vi "HFRR ADV v06 new software.vi"() -> ()   [LabVIEW 2025] (continued)
                        n2282 = local read "Set Temp"() -> (w3342:dbl)
                        n2283 = Number To Fractional String(number=w3342, precision (6)=i16 2) -> (F-format string=w3343:string)  [unwired: 2 in]
                        n2284 = Concatenate Strings("Set Temperature [deg C] :" ("Content"), w3343) -> (w3345:string)
                        n2285 = local read "EVENT LOG"() -> (w3347:string)
                        n2286 = call "Event Log.vi"("Content"=w3345, "EVENT LOG"=w3347) -> ("EVENT LOG"=w3346:string)  [unwired: 8 in, 1 out]
                        n2287 = local write "EVENT LOG"(w3346) -> ()
                      }
                      frame #28 {
                        n2288 = Wait (ms)(milliseconds to wait=u32 50) -> ()  [unwired: 1 out]
                      }
                      frame #29 {
                        n2289 = local read "Set Rh"() -> (w3350:dbl)
                        n2290 = Number To Fractional String(number=w3350, precision (6)=i16 2) -> (F-format string=w3351:string)  [unwired: 2 in]
                        n2291 = Concatenate Strings("Set Humidity [%RH] :" ("Content"), w3351) -> (w3353:string)
                        n2292 = local read "EVENT LOG"() -> (w3355:string)
                        n2293 = call "Event Log.vi"("Content"=w3353, "EVENT LOG"=w3355) -> ("EVENT LOG"=w3354:string)  [unwired: 8 in, 1 out]
                        n2294 = local write "EVENT LOG"(w3354) -> ()
                      }
                      frame #30 {
                        n2295 = Wait (ms)(milliseconds to wait=u32 50) -> ()  [unwired: 1 out]
                      }
                      frame #31 {
                        n2296 = local read "test time"() -> (w3358:dbl)
                        n2297 = Number To Fractional String(number=w3358, precision (6)=i16 1) -> (F-format string=w3359:string)  [unwired: 2 in]
                        n2298 = Concatenate Strings("Test Duration [mins] :" ("Content"), w3359) -> (w3361:string)
                        n2299 = local read "EVENT LOG"() -> (w3363:string)
                        n2300 = call "Event Log.vi"("Content"=w3361, "EVENT LOG"=w3363) -> ("EVENT LOG"=w3362:string)  [unwired: 8 in, 1 out]
                        n2301 = local write "EVENT LOG"(w3362) -> ()
                      }
                      frame #32 {
                        w3364 = dbl[] [] ("History Data")
                        w3365 = cluster{"y":dbl, dbl, "y":dbl}[] [] ("History Data")
                        w3366 = FALSE ("Visible")
                        n2302 = property on="Stroke ( mm )" class="WFChart (strict)"("History Data"=w3365) -> ()  [unwired: 2 in, 2 out]
                        n2303 = property on="Humidity ( %RH )" class="WFChart (strict)"("History Data"=w3364) -> ()  [unwired: 2 in, 2 out]
                        n2304 = property on="Temperature ( Deg C )" class="WFChart (strict)"("History Data"=w3364) -> ()  [unwired: 2 in, 2 out]
                        n2305 = property on="Electrical Contact Resistance ( % )" class="WFChart (strict)"("History Data"=w3364) -> ()  [unwired: 2 in, 2 out]
                        n2306 = property on="Coefficient of Friction" class="WFChart (strict)"("History Data"=w3364) -> ()  [unwired: 2 in, 2 out]
                        n2307 = property on="Frictional Force ( N )" class="WFChart (strict)"("History Data"=w3364) -> ()  [unwired: 2 in, 2 out]
                        n2308 = property on="Coefficient of Friction" class="WFChart (strict)"("History Data"=w3364) -> ()  [unwired: 2 in, 2 out]
                        n2309 = property on="Frictional Force ( N )" class="WFChart (strict)"("History Data"=w3364) -> ()  [unwired: 2 in, 2 out]
                        n2310 = property on="Electrical Contact Resistance ( % )" class="WFChart (strict)"("History Data"=w3364) -> ()  [unwired: 2 in, 2 out]
                        n2311 = property on="Humidity ( %RH )" class="WFChart (strict)"("History Data"=w3364) -> ()  [unwired: 2 in, 2 out]
                        n2312 = property on="Stroke ( mm )" class="WFChart (strict)"("History Data"=w3365) -> ()  [unwired: 2 in, 2 out]
                        n2313 = property on="Temperature ( Deg C )" class="WFChart (strict)"("History Data"=w3364) -> ()  [unwired: 2 in, 2 out]
                        n2314 = property on="Service Password Log" class="Str"("Visible"=w3366) -> ()  [unwired: 2 in, 2 out]
                        n2315 = property on="Password 3" class="Clust (strict)"("Visible"=w3366) -> ()  [unwired: 2 in, 2 out]
                      }
                    }
                    "TEST FILE NAM,E SAVED" <- TRUE ("TEST FILE NAM,E SAVED")
                  }
                }
              }
            }
          }
        }
        n2316 = case shown="True" w2670 {
          frame False {
            n2317 = local write "tfalg"(0.0 ("tfalg")) -> ()
          }
          frame True {
            n2318 = local read "tfalg"() -> (w2815:dbl)
            n2319 = Equal?(x=w2815, y=0.0) -> (x = y?=w2816:bool)
            n2320 = case shown="True" w2816 {
              frame False {
              }
              frame True {
                n2321 = local read "Total No. of Tests"() -> (w2819:dbl)
                n2322 = local write "tfalg"(1.0 ("tfalg")) -> ()
                n2323 = local write "acq 2"(FALSE ("acq 2")) -> ()
                n2324 = Wait (ms)(milliseconds to wait=u32 200) -> ()  [unwired: 1 out]
                n2325 = Increment(x=w2819) -> (x+1=w2818:dbl)
                n2326 = local write "Total No. of Tests"(w2818) -> ()
              }
            }
          }
        }
        n2327 = local write "Test \nStatus"(w2676) -> ()
        n2328 = local write "Save"(w2676) -> ()
        n2329 = local read "Main Tab"() -> (w2633:T2)
        n2330 = case shown="True" w2657 {
          tunnel: [FALSE ("RUN") TRUE ("RUN")] -> w2656
          tunnel: [_ 1] -> w2649
          frame False {
          }
          frame True {
          }
        }
        n2331 = In Range and Coerce(upper limit=w2664, x=w2637, lower limit=w2663) -> (In Range?=w2655:bool)  [unwired: 1 out]
        n2332 = In Range and Coerce(upper limit=w2661, x=w2636, lower limit=w2662) -> (In Range?=w2653:bool)  [unwired: 1 out]
        n2333 = case shown="True" w2669 {
          frame False {
            n2334 = local read "Rt 3"() -> (w2797:bool)
            n2335 = case shown="True" w2797 {
              frame False {
              }
              frame True {
                n2336 = local write "Rt 3"(FALSE ("Rt 3")) -> ()
                n2337 = local write "Json End Flg"(TRUE ("Upld AR 2")) -> ()
              }
            }
            "Rt" <- TRUE ("Rt")
            "Rt 2" <- FALSE ("Rt")
          }
          frame True {
            n2338 = local read "Rt"() -> (w2804:bool)
            n2339 = local write "Rt 2"(TRUE ("Rt 2")) -> ()
            n2340 = case shown="True" w2804 {
              frame False {
              }
              frame True {
                w2805 = TRUE ("Upld AR 2")
                n2341 = local write "Rt"(FALSE ("Rt")) -> ()
                n2342 = local write "Upld AR"(w2805) -> ()
                n2343 = local write "Json St Flg"(w2805) -> ()
              }
            }
            "Rt 3" <- TRUE ("Rt 3")
          }
        }
        n2344 = case shown="True" w2655 {
          tunnel: [FALSE ("RUN") TRUE ("RUN")] -> w2654
          tunnel: [_ 2] -> w2648
          frame False {
          }
          frame True {
          }
        }
        n2345 = case shown="True" w2653 {
          tunnel: [FALSE ("RUN") TRUE ("RUN")] -> w2652
          tunnel: [_ 3] -> w2647
          frame False {
          }
          frame True {
          }
        }
        n2346 = case shown="\"Acquire\"" w2633 {
          tunnel: w2635 -> [_ w2866]
          frame Default {
            w2865 = 0.0 ("output")
            n2347 = local write "PID-out"(w2865) -> ()
            n2348 = local write "Frequency ( Hz )"(w2865) -> ()
          }
          frame "Acquire" {
            n2349 = stacked-sequence {
              frame #0 {
                n2350 = local read "Auto Start Test"() -> (w2868:bool)
                n2351 = case shown="True" w2868 {
                  tunnel: "RUN" -> [w2889 w2892]
                  tunnel: [w2889 w2891] -> w2869
                  frame False {
                  }
                  frame True {
                    n2352 = local read "Auto Start Temp"() -> (w2890:bool)
                    n2353 = Or(x=w2892, y=w2890) -> (x .or. y?=w2891:bool)
                  }
                }
                n2354 = local read "clk"() -> (w2888:dbl)
                n2355 = local read "Save"() -> (w2884:bool)
                n2356 = Equal?(x=w2888, y=0.0) -> (x = y?=w2885:bool)
                n2357 = And(x=w2885, y=w2884) -> (x .and. y?=w2886:bool)
                n2358 = Not(x="Engage") -> (.not. x?=w2875:bool)
                n2359 = case shown="False" w2869 {
                  tunnel: [0.0 w2910] -> w2871
                  frame False {
                    (unwired) TRUE ("Visible")
                    n2360 = local read "Auto Start Test"() -> (w2896:bool)
                    n2361 = local write "Start Time"(TRUE ("Start Time")) -> ()
                    n2362 = property on="Stroke 2" class="DigNum (strict)"("Visible"=FALSE) -> ()  [unwired: 2 in, 2 out]
                    n2363 = case shown="False" w2896 {
                      frame False {
                        n2364 = property on="Heater Button" class="Bool (strict)"("DisabledEnum"=T13."Enabled" ("Disabled")) -> ()  [unwired: 2 in, 2 out]
                        n2365 = property on="Humidity" class="Bool (strict)"("DisabledEnum"=T13."Enabled" ("Disabled")) -> ()  [unwired: 2 in, 2 out]
                      }
                      frame True {
                      }
                    }
                    n2366 = case shown="False" "TestCompFlg" {
                      frame False {
                        n2367 = local read "StartFlg"() -> (w2904:bool)
                        n2368 = case shown="True" w2904 {
                          frame False {
                          }
                          frame True {
                            n2369 = flat-sequence {
                              frame #0 {
                                n2370 = local read "EVENT LOG"() -> (w2906:string)
                                n2371 = call "Event Log.vi"("Content"="Test was interrupted", "EVENT LOG"=w2906) -> ("EVENT LOG"=w2907:string)  [unwired: 8 in, 1 out]
                                n2372 = local write "EVENT LOG"(w2907) -> ()
                              }
                              frame #1 {
                                w2909 = FALSE ("StartFlg")
                                n2373 = property on="Heater Button" class="Bool (strict)"("Val(Sgnl)"=FALSE ("Value (Signaling)")) -> ()  [unwired: 2 in, 2 out]
                                n2374 = local write "Heater Button"(w2909) -> ()
                                n2375 = local write "StartFlg"(w2909) -> ()
                                n2376 = local write "Humidity"(w2909) -> ()
                              }
                            }
                          }
                        }
                      }
                      frame True {
                      }
                    }
                    n2377 = local write "String 14"("Test will autostart once parameters reach the set value." ("String 14")) -> ()
                  }
                  frame True {
                    (unwired) FALSE ("Visible")
                    n2378 = property on="Stroke 2" class="DigNum (strict)"("Visible"=TRUE) -> ()  [unwired: 2 in, 2 out]
                    n2379 = property on="STOP 2" class="Bool (strict)"("Disabled"=u8 2) -> ()  [unwired: 2 in, 2 out]
                    n2380 = local write "String 14"(" Running....." ("String 14")) -> ()
                    n2381 = property on="Heater Button" class="Bool (strict)"("DisabledEnum"=T13."Disabled and Grayed Out" ("Disabled")) -> ()  [unwired: 2 in, 2 out]
                    n2382 = property on="Humidity" class="Bool (strict)"("DisabledEnum"=T13."Disabled and Grayed Out" ("Disabled")) -> ()  [unwired: 2 in, 2 out]
                    n2383 = case shown="True" "Start Time" {
                      selector: "Start Time" -> [_ w2929]
                      frame False {
                      }
                      frame True {
                        n2384 = Not(x=w2929) -> (.not. x?=w2928:bool)
                        n2385 = local write "Start Time"(w2928) -> ()
                        n2386 = local read "EVENT LOG"() -> (w2930:string)
                        n2387 = call "Event Log.vi"("Content"="Test in progress", "EVENT LOG"=w2930) -> ("EVENT LOG"=w2932:string)  [unwired: 8 in, 1 out]
                        n2388 = local write "EVENT LOG"(w2932) -> ()
                      }
                    }
                    n2389 = disable-structure shown="Enabled" {
                      disable-tunnel: [w2921 w2927] -> w2910
                      frame Disabled {
                        n2390 = local read "Set Hz"() -> (w2924:dbl)
                        n2391 = call <vilib>:"Uniform White Noise Waveform.vi"() -> ("signal out"=w2923:waveform(dbl))  [unwired: 10 in, 1 out]
                        n2392 = Random Number (0-1)() -> (number: 0 to 1=w2920:dbl)
                        n2393 = Add(x=w2924, y=w2923) -> (x+y=w2922:waveform(dbl))
                        n2394 = Multiply(x=ext 0.01 ("y"), y=w2920) -> (x*y=w2918:ext)
                        n2395 = Multiply(x=w2922, y=w2918) -> (x*y=w2921:waveform(ext))
                      }
                      frame Enabled {
                        n2396 = call-poly <vilib>:"Random Number (Range).vi"("lower bound (0)"=49.5, "upper bound (100)"=50.5) -> ("number"=w2927:dbl)  [unwired: 9 in]
                      }
                    }
                    "StartFlg" <- TRUE ("StartFlg")
                  }
                }
                n2397 = case shown="True" w2886 {
                  frame False {
                  }
                  frame True {
                    n2398 = local write "clk"(10.0 ("clk")) -> ()
                    n2399 = Get Date/Time In Seconds() -> (seconds since 1Jan1904=w2935:timestamp)
                    n2400 = To Double Precision Float(number=w2935) -> (double precision float=w2933:dbl)
                    n2401 = local write "acq timer"(w2933) -> ()
                    n2402 = local write "act save time"(w2933) -> ()
                  }
                }
                n2403 = call "Elapsed Time"("Time Target (s)"="Countdown", "Reset"=w2875) -> ("Elapsed Time (s)"=w2880:dbl, "Time has Elapsed"=w2878:bool)  [unwired: 10 in, 6 out]
                "Countdown 2" <- w2880
                n2404 = Subtract(x=w2880, y=2.0) -> (x-y=w2883:dbl)
                n2405 = Less?(x=w2883, y="Countdown") -> (x < y?=w2881:bool)
                n2406 = And(x=w2881, y=w2878) -> (x .and. y?=w2877:bool)
                n2407 = case shown="True" w2877 {
                  frame False {
                  }
                  frame True {
                    (unwired) dbl[] [] ("History Data")
                    n2408 = local write "Engage"(FALSE ("Engage")) -> ()
                    n2409 = local write "RUN"(TRUE ("RUN")) -> ()
                    n2410 = local read "Humidity ( %RH )"() -> (→"Rh Before":dbl)
                  }
                }
                n2411 = local read "Test \nStatus"() -> (w2873:bool)
                n2412 = Select(t=w2871, s=w2873, f=0.0) -> (s? t:f=w2872:dbl)
                n2413 = local write "Frequency ( Hz )"(w2872) -> ()
              }
              frame #1 {
                w2958 = 1000000.0 ("x")
                # "HC;1/0\nST;VALUE"
                # "Elapsed time\ncof\nstroke\nAir temp\nTemp\nHumidity"
                # "acq timer\n\nact save time"
                # "convert to microseconds"
                n2414 = local read "COUNT"() -> (w2941:i32)
                n2415 = local read "Rate"() -> (w2954:dbl)
                n2416 = Divide(x=w2958, y=w2954) -> (x/y=w2959:dbl)
                n2417 = Greater Or Equal?(x=w2941, y=250) -> (x >= y?=w2940:bool)
                n2418 = Get Date/Time In Seconds() -> (seconds since 1Jan1904=w2961:timestamp)
                n2419 = case shown="True" w2940 {
                  frame False {
                    n2420 = local read "COUNT"() -> (w2962:i32)
                    n2421 = Increment(x=w2962) -> (x+1=w2963:i32)
                    n2422 = local write "COUNT"(w2963) -> ()
                  }
                  frame True {
                    n2423 = local write "COUNT"(0 ("COUNT")) -> ()
                  }
                }
                n2424 = local read "Samplingtime 2"() -> (w2939:dbl)
                n2425 = local read "act save time"() -> (w2956:dbl)
                n2426 = Divide(x=w2959, y=w2958) -> (x/y=w2957:dbl)
                n2427 = To Double Precision Float(number=w2961) -> (double precision float=w2950:dbl)
                n2428 = Add(x=w2956, y=w2939) -> (x+y=w2955:dbl)
                n2429 = local read "acq timer"() -> (w2960:dbl)
                n2430 = local read "COUNT"() -> (w2943:i32)
                n2431 = Greater Or Equal?(x=w2950, y=w2955) -> (x >= y?=w2938:bool)
                n2432 = Multiply(x=w2957, y=w2943) -> (x*y=w2949:dbl)
                n2433 = Subtract(x=w2950, y=w2960) -> (x-y=w2952:dbl)
                n2434 = local read "Save"() -> (w2953:bool)
                n2435 = Add(x=w2952, y=w2949) -> (x+y=w2936:dbl)
                "Elapsed time 3" <- w2936
                n2436 = And(x=w2938, y=w2953) -> (x .and. y?=w2951:bool)
                n2437 = Divide(x=w2936, y=60.0) -> (x/y=w2947:dbl)
                n2438 = local read "Test \nStatus"() -> (w2937:bool)
                n2439 = local read "clk"() -> (w2944:dbl)
                n2440 = Equal?(x=w2944, y=10.0) -> (x = y?=w2946:bool)
                n2441 = case shown="True" w2951 {
                  tunnel: w2950 -> [_ w3072]
                  tunnel: [FALSE ("Boolean 2") TRUE ("Boolean 2")] -> _
                  frame False {
                  }
                  frame True {
                    w3026 = ";" ("Substring")
                    # "Pid out/\nFreq response value"
                    n2442 = local write "act save time"(w3072) -> ()
                    n2443 = local read "FILE"() -> (w3020:string)
                    n2444 = call "file check.vi"("file name in"=w3020) -> ("error out"=w3023:errorcluster, "file name out"=w3018:string)  [unwired: 9 in]
                    n2445 = call "FILE PATH CREATION.vi"("error in"=w3023, "FILE NAME :"=w3018) -> ("FILE OUT"=w3021:path)  [unwired: 8 in, 1 out]
                    n2446 = Concatenate Strings(w3018, ".dgf" ("Substring")) -> (w3022:string)
                    n2447 = local read "FF 2"() -> (→"Frictional Force ( N )" →"Frictional Force ( N )":dbl)
                    n2448 = Build Path(base path=w3021, name or relative path=w3022) -> (appended path=w3017:path)
                    n2449 = local read "COF 2"() -> (w3031:dbl)
                    "cof" <- w3031
                    "Coefficient of Friction" <- w3031
                    "COF 4" <- w3031
                    "Coefficient of Friction" <- w3031
                    n2450 = local read "LVDT STROKE"() -> (w3015:dbl)
                    n2451 = local read "Add up Stroke"() -> (w3013:dbl)
                    n2452 = local read "TEMP"() -> (w3034:dbl)
                    "Temp" <- w3034
                    "Temperature ( Deg C )" <- w3034
                    n2453 = local read "Humidity ( %RH )"() -> (w3033:dbl)
                    "Humidity ( %RH )" <- w3033
                    "Humidity ( %RH )" <- w3033
                    n2454 = local read "Frequency ( Hz )"() -> (w3040:dbl)
                    n2455 = local read "Elapsed time"() -> (w3065:dbl)
                    n2456 = local read "AIR TEMP"() -> (w3038:dbl)
                    n2457 = local read "PID-out"() -> (w3043:dbl)
                    n2458 = Subtract(x=w3015, y=w3013) -> (x-y=w3014:dbl)
                    n2459 = Absolute Value(x=w3014) -> (abs(x)=w3012:dbl)
                    n2460 = local write "Temperature ( Deg C )"(w3034) -> ()
                    n2461 = Number To Fractional String(number=w3012, width (-)=i16 9 ("precision (6)"), precision (6)=i16 6) -> (F-format string=w3058:string)  [unwired: 1 in]
                    n2462 = Number To Fractional String(number=w3038, width (-)=i16 9 ("precision (6)"), precision (6)=i16 3) -> (F-format string=w3057:string)  [unwired: 1 in]
                    n2463 = Number To Fractional String(number=w3034, width (-)=i16 9 ("precision (6)"), precision (6)=i16 3) -> (F-format string=w3054:string)  [unwired: 1 in]
                    n2464 = Number To Fractional String(number=w3033, width (-)=i16 9 ("precision (6)"), precision (6)=i16 3) -> (F-format string=w3051:string)  [unwired: 1 in]
                    n2465 = Number To Fractional String(number=0.0, width (-)=i16 9 ("precision (6)"), precision (6)=i16 3) -> (F-format string=w3048:string)  [unwired: 1 in]
                    n2466 = Number To Fractional String(number=w3043, width (-)=i16 9 ("precision (6)"), precision (6)=i16 3) -> (F-format string=w3044:string)  [unwired: 1 in]
                    n2467 = Number To Fractional String(number=w3040, width (-)=i16 9 ("precision (6)"), precision (6)=i16 3) -> (F-format string=w3039:string)  [unwired: 1 in]
                    n2468 = Number To Fractional String(number=w3031, width (-)=i16 9 ("precision (6)"), precision (6)=i16 6) -> (F-format string=w3066:string)  [unwired: 1 in]
                    n2469 = Number To Fractional String(number=w3065, width (-)=i16 14 ("precision (6)"), precision (6)=i16 3) -> (F-format string=w3067:string)  [unwired: 1 in]
                    n2470 = Bundle("y"=1.02, w3012, "y"=0.98) -> (w3032:cluster{"y":dbl, dbl, "y":dbl})  [unwired: 1 in]
                    n2471 = Number To Fractional String(number="Ambient Humidity :", width (-)=i16 9 ("precision (6)"), precision (6)=i16 6) -> (F-format string=w3024:string)  [unwired: 1 in]
                    n2472 = local read "RUN"() -> (w3030:bool)
                    n2473 = case shown="True" w3030 {
                      tunnel: w3032 -> [_ w3077]
                      tunnel: w3012 -> [_ w3076]
                      tunnel: w3012 -> [_ w3074]
                      tunnel: w3012 -> [_ w3075]
                      frame False {
                      }
                      frame True {
                        "Stroke ( mm )" <- w3077
                        "Stroke ( mm )" <- w3077
                        "Stroke 4" <- w3076
                        "Stroke 3" <- w3074
                        "Stroke 2" <- w3075
                        "measured_stroke" <- w3074
                      }
                    }
                    n2474 = Concatenate Strings(w3067, w3026, w3066, w3026, w3058, w3026, w3057, w3026, w3054, w3026, w3051, w3026, w3048, w3026, w3044, w3026, w3039, w3026, w3024, "\r") -> (w3064:string)
                    n2475 = call <vilib>:"Write Characters To File.vi"("append to file? (new file:F)"=TRUE, "character string"=w3064, "file path (dialog if empty)"=w3017) -> ()  [unwired: 2 in, 1 out]
                    "refresh flag" <- TRUE ("refresh flag")
                  }
                }
                n2476 = case shown="True" w2937 {
                  tunnel: w2947 -> [_ w2973]
                  tunnel: w2952 -> [_ w2983]
                  tunnel: [0.0 w2979] -> _
                  tunnel: w2946 -> [_ w2978]
                  tunnel: [0.0 w2977] -> _
                  tunnel: w2936 -> [_ w2977]
                  tunnel: w2950 -> [w2966 _]
                  frame False {
                    n2477 = local write "acq timer"(w2966) -> ()
                    n2478 = local write "Test Duration Status"(0.0 ("Test Duration Status")) -> ()
                  }
                  frame True {
                    n2479 = local read "Set Hz"() -> (w2980:dbl)
                    n2480 = local write "Elapsed time"(w2973) -> ()
                    n2481 = local read "test time"() -> (w2972:dbl)
                    n2482 = Multiply(x=w2983, y=w2980) -> (x*y=w2982:dbl)
                    n2483 = case shown="False" w2978 {
                      tunnel: w2982 -> [w2984 _]
                      tunnel: [w2984 1.0] -> w2979
                      frame False {
                        n2484 = local write "Cycles elapsed"(w2984) -> ()
                      }
                      frame True {
                      }
                    }
                    n2485 = Greater?(x=w2973, y=w2972) -> (0:w2981:bool)
                    n2486 = Subtract(x=w2972, y=w2973) -> (x-y=w2971:dbl)
                    "time" <- w2971
                    n2487 = Multiply(x=w2971, y=60.0) -> (x*y=w2970:dbl)
                    n2488 = local write "Time Remaining"(w2970) -> ()
                    n2489 = local write "Remaining Time"(w2970) -> ()
                    n2490 = case shown="True" w2981 {
                      frame False {
                      }
                      frame True {
                        n2491 = stacked-sequence {
                          frame #0 {
                            w2989 = T13."Enabled" ("Disabled")
                            w2988 = FALSE ("TEST FILE NAM,E SAVED")
                            w2990 = "" ("FILE")
                            w2991 = TRUE ("Visible")
                            n2492 = local write "Humidity"(FALSE ("Humidity")) -> ()
                            n2493 = local write "RUN"(FALSE ("OK Button 2")) -> ()
                            n2494 = local write "Heater Button"(FALSE ("Heater Button")) -> ()
                            n2495 = local write "Auto Start Test"(FALSE ("Auto Start Test")) -> ()
                            n2496 = local write "TestCompFlg"(TRUE ("StpFlg")) -> ()
                            n2497 = local read "Humidity ( %RH )"() -> (→"Rh After":dbl)
                            n2498 = property on="STOP 2" class="Bool (strict)"("Disabled"=u8 0) -> ()  [unwired: 2 in, 2 out]
                            n2499 = local read "EVENT LOG"() -> (w2996:string)
                            n2500 = call "Event Log.vi"("Content"="Test Completed", "EVENT LOG"=w2996) -> ("EVENT LOG"=w2995:string)  [unwired: 8 in, 1 out]
                            n2501 = property on="RUN" class="Bool (strict)"("Visible"=w2991) -> ()  [unwired: 2 in, 2 out]
                            n2502 = property on="Auto Start Test" class="Bool (strict)"("Visible"=w2991) -> ()  [unwired: 2 in, 2 out]
                            n2503 = local write "Batch Ref Num :"(w2990) -> ()
                            n2504 = local write "FILE"(w2990) -> ()
                            n2505 = local write "EVENT LOG"(w2995) -> ()
                            n2506 = local write "TEST FILE NAM,E SAVED"(w2988) -> ()
                            n2507 = local write "Fuel Discription :"(w2990) -> ()
                            n2508 = local write "START TEMP"(w2988) -> ()
                            n2509 = local write "Remarks :"(w2990) -> ()
                            n2510 = local write "Main Dashboard Buttons"(T1."Imaging" ("Main Dashboard Buttons")) -> ()
                            n2511 = local write "Main Tab"(T2."Adv Scar" ("Main Tab")) -> ()
                            n2512 = property on="FRICVALZ 2" class="Bool (strict)"("DisabledEnum"=w2989) -> ()  [unwired: 2 in, 2 out]
                            n2513 = property on="FRICVALZ 3" class="Bool (strict)"("DisabledEnum"=w2989) -> ()  [unwired: 2 in, 2 out]
                            n2514 = property on="FRICVALZ 4" class="Bool (strict)"("DisabledEnum"=w2989) -> ()  [unwired: 2 in, 2 out]
                          }
                          frame #1 {
                            n2515 = Wait (ms)(milliseconds to wait=u32 1500) -> ()  [unwired: 1 out]
                          }
                          frame #2 {
                            n2516 = local write "Command"("VC;0") -> ()
                          }
                          frame #3 {
                            n2517 = Wait (ms)(milliseconds to wait=u32 1500) -> ()  [unwired: 1 out]
                          }
                          frame #4 {
                            n2518 = local write "Command"("VC;0") -> ()
                          }
                          frame #5 {
                            n2519 = Wait (ms)(milliseconds to wait=u32 1500) -> ()  [unwired: 1 out]
                          }
                          frame #6 {
                            n2520 = local write "Command"("ST;0") -> ()
                          }
                          frame #7 {
                            n2521 = local write "measured_stroke"(0.0 ("measured_stroke")) -> ()
                            n2522 = Wait (ms)(milliseconds to wait=u32 1500) -> ()  [unwired: 1 out]
                          }
                          frame #8 {
                            n2523 = local write "Command"("HE;0") -> ()
                          }
                        }
                      }
                    }
                    n2524 = Divide(x=w2973, y=w2972) -> (x/y=w2976:dbl)
                    n2525 = Multiply(x=w2976, y=100.0) -> (x*y=w2974:dbl)
                    n2526 = local write "Test Duration Status"(w2974) -> ()
                  }
                }
              }
              frame #2 {
                n2527 = case shown="True" "Heater Button" {
                  tunnel: [0.0 ("output") w3100] -> w3078
                  frame False {
                    w3081 = TRUE ("tmpchk")
                    n2528 = local read "TEMP"() -> (w3082:dbl)
                    n2529 = local write "Temp ini"(w3082) -> ()
                    n2530 = local write "Reset 4"(w3081) -> ()
                    n2531 = local write "tmpchk"(w3081) -> ()
                    n2532 = local write "reinit"(TRUE ("reinit")) -> ()
                    n2533 = local write "manual temp log"(TRUE ("manual temp log")) -> ()
                  }
                  frame True {
                    # "Logic to turn off\nthe heater when \ntemp is not rising.\nTime - 60 sec\nDelta t- 5°c"
                    n2534 = local read "Temp ini"() -> (w3089:dbl)
                    n2535 = local read "Auto Start Test"() -> (w3085:bool)
                    n2536 = Less?(x=w3089, y=53.0) -> (x < y?=w3087:bool)
                    n2537 = case shown="False" w3085 {
                      frame False {
                        n2538 = local read "Set Temp"() -> (w3109:dbl)
                        n2539 = local read "TEMP"() -> (w3108:dbl)
                        n2540 = Subtract(x=w3109, y=w3108) -> (x-y=w3107:dbl)
                        n2541 = Absolute Value(x=w3107) -> (abs(x)=w3106:dbl)
                        n2542 = Less?(x=w3106, y=0.5) -> (x < y?=w3104:bool)
                        n2543 = case shown="True" w3104 {
                          tunnel: "manual temp log" -> [_ w3110]
                          frame False {
                          }
                          frame True {
                            n2544 = case shown="True" w3110 {
                              selector: w3110 -> [_ w3111]
                              frame False {
                              }
                              frame True {
                                # "#Event log"
                                n2545 = Not(x=w3111) -> (.not. x?=w3112:bool)
                                n2546 = local write "manual temp log"(w3112) -> ()
                                n2547 = local read "EVENT LOG"() -> (w3115:string)
                                n2548 = call "Event Log.vi"("Content"="Target Temperature reached", "EVENT LOG"=w3115) -> ("EVENT LOG"=w3114:string)  [unwired: 8 in, 1 out]
                                n2549 = local write "EVENT LOG"(w3114) -> ()
                              }
                            }
                          }
                        }
                      }
                      frame True {
                        n2550 = local write "manual temp log"(TRUE ("manual temp log")) -> ()
                      }
                    }
                    n2551 = And(x="tmpchk", y=w3087) -> (x .and. y?=w3090:bool)
                    n2552 = case shown="True" w3090 {
                      frame False {
                      }
                      frame True {
                        n2553 = call "Elapsed Time8"("Time Target (s)"=300.0, "Reset"="Reset 4") -> ("Time has Elapsed"=w3117:bool)  [unwired: 10 in, 7 out]
                        n2554 = flat-sequence {
                          tunnel: w3117 -> [_]
                          frame #0 {
                            n2555 = local write "Reset 4"(FALSE ("Reset 4")) -> ()
                          }
                        }
                        n2556 = case shown="True" w3117 {
                          frame False {
                          }
                          frame True {
                            n2557 = local read "Temp ini"() -> (w3124:dbl)
                            n2558 = Add(x=w3124, y=5.0) -> (x+y=w3122:dbl)
                            n2559 = local read "TEMP"() -> (w3125:dbl)
                            n2560 = Greater?(x=w3125, y=w3122) -> (0:w3123:bool)
                            n2561 = case shown="False" w3123 {
                              frame False {
                                n2562 = local write "Heater Button"(FALSE ("Heater Button")) -> ()
                              }
                              frame True {
                                n2563 = local write "tmpchk"(FALSE ("tmpchk")) -> ()
                              }
                            }
                          }
                        }
                      }
                    }
                    n2564 = local read "Set Temp"() -> (w3098:dbl)
                    n2565 = local read "TEMP"() -> (w3092:dbl)
                    n2566 = call-poly <vilib>:"PID.vi"("reinitialize? (F)"="reinit", "dt (s)"=-1.0, "process variable"=w3092, "setpoint"=w3098) -> ("output"=w3095:dbl)  [unwired: 6 in, 1 out]
                    n2567 = Subtract(x=w3098, y=w3092) -> (x-y=w3099:dbl)
                    n2568 = Add(x=w3098, y=0.5) -> (x+y=w3096:dbl)
                    n2569 = Greater Or Equal?(x=w3092, y=w3096) -> ()  [unwired: 1 out]
                    n2570 = Select(t=0.0, s=FALSE, f=w3095) -> (s? t:f=w3094:dbl)
                    "PID output" <- w3094
                    n2571 = flat-sequence {
                      tunnel: w3094 -> [w3128]
                      tunnel: [w3128] -> w3100
                      frame #0 {
                        n2572 = local write "reinit"(FALSE ("reinit")) -> ()
                      }
                    }
                    n2573 = Bundle(w3099, "output"=w3094, "TEMP"=w3092) -> ()  [unwired: 1 in, 1 out]
                  }
                }
                "PID-out" <- w3078
              }
              frame #3 {
                n2574 = local read "TEMP"() -> (w3130:dbl)
                n2575 = Greater Or Equal?(x=w3130, y="Set Temp 2") -> (x >= y?=w3135:bool)
                n2576 = case shown="True" w3135 {
                  tunnel: [FALSE TRUE] -> w3133
                  frame False {
                  }
                  frame True {
                  }
                }
                "Status 13" <- w3133
                n2577 = And(x=w3133, y="trip1 8") -> (x .and. y?=w3132:bool)
                n2578 = case shown="True" w3132 {
                  frame False {
                    n2579 = local write "Heater Trip Temp"(TRUE ("Heater Trip Temp")) -> ()
                  }
                  frame True {
                    w3138 = FALSE ("OK Button 2")
                    n2580 = case shown="True" "Heater Trip Temp" {
                      selector: "Heater Trip Temp" -> [_ w3140]
                      frame False {
                      }
                      frame True {
                        n2581 = Not(x=w3140) -> (.not. x?=w3139:bool)
                        n2582 = local read "EVENT LOG"() -> (w3143:string)
                        n2583 = local write "Heater Trip Temp"(w3139) -> ()
                        n2584 = call "Event Log.vi"("Content"="Heater Trip", "EVENT LOG"=w3143) -> ("EVENT LOG"=w3142:string)  [unwired: 8 in, 1 out]
                        n2585 = local write "EVENT LOG"(w3142) -> ()
                      }
                    }
                    n2586 = local write "RUN"(w3138) -> ()
                    n2587 = property on="Auto Start Test" class="Bool (strict)"("Value"=w3138) -> ()  [unwired: 2 in, 2 out]
                    n2588 = local write "Heater Button"(w3138) -> ()
                  }
                }
              }
            }
            n2589 = case shown="False" w2866 {
              frame False {
                n2590 = disable-structure shown="Disabled" {
                  frame Disabled {
                    n2591 = stacked-sequence {
                      frame #0 {
                        n2592 = local write "RUN"(FALSE ("OK Button 2")) -> ()
                      }
                      frame #1 {
                      }
                    }
                  }
                  frame Enabled {
                  }
                }
              }
              frame True {
              }
            }
          }
        }
        n2593 = local read "airtempflg"() -> (w2658:bool)
        n2594 = Or(x=w2658, y=w2656) -> (x .or. y?=w2659:bool)
        n2595 = Insert Into Array(array=string[] ["Air Temperature has reached set value,", "Humidity has reached set value,", "Sample Temperaturehas reached set value,", ""], index=0, new element="") -> (w2644:string[])
        n2596 = Build Array(w2649, w2648, w2647) -> (w2645:i32[])
        n2597 = disable-structure shown="Disabled" {
          disable-tunnel: w2659 -> [w2736 _]
          disable-tunnel: w2654 -> [w2735 _]
          disable-tunnel: w2652 -> [w2734 _]
          frame Disabled {
            n2598 = Compound Arithmetic op=AND(w2736, w2735, w2734) -> ()  [unwired: 1 out]
            n2599 = case shown="True" {
              selector: _ -> [_ _]
              frame False {
              }
              frame True {
                w2737 = FALSE ("autostrtflg")
                n2600 = local write "RUN"(TRUE ("RUN")) -> ()
                n2601 = local write "autostrtflg"(w2737) -> ()
                n2602 = local write "autostart"(w2737) -> ()
                n2603 = local write "String 14"(" Running....." ("String 14")) -> ()
              }
            }
          }
          frame Enabled {
          }
        }
        n2604 = for {
          tunnel: w2645 -> [w2787] mode=indexing
          tunnel: w2644 -> [w2786]
          shift-right: [w2783] -> w2643
          shift-left: "" -> [w2785]
          n2605 = Index Array(array=w2786, index=w2787) -> (element=w2784:string)
          n2606 = Concatenate Strings(w2784, w2785) -> (w2783:string)
        }
        n2607 = local write "autostart 2"(w2643) -> ()
        n2608 = local read "Reset Graph"() -> (w2632:bool)
        n2609 = case shown="True" w2632 {
          selector: w2632 -> [_ w2686]
          frame False {
          }
          frame True {
            w2700 = 0.0 ("X Scale.Range:Maximum")
            n2610 = Not(x=w2686) -> (.not. x?=w2685:bool)
            n2611 = local write "Reset Graph"(w2685) -> ()
            n2612 = property on="Electrical Contact Resistance ( % )" class="WFChart (strict)"("XScale.Maximum"=600.0 ("X Scale.Range:Maximum"), "XScale.Minimum"=0.0 ("X Scale.Range:Minimum"), "YScale.Maximum"=100.0 ("Y Scale.Range:Maximum"), "YScale.Minimum"=0.0 ("Y Scale.Range:Minimum")) -> ()  [unwired: 2 in, 2 out]
            n2613 = property on="Frictional Force ( N )" class="WFChart (strict)"("XScale.Maximum"=600.0 ("X Scale.Range:Maximum"), "XScale.Minimum"=0.0 ("X Scale.Range:Minimum"), "YScale.Maximum"=100.0 ("Y Scale.Range:Maximum"), "YScale.Minimum"=0.0 ("Y Scale.Range:Minimum")) -> ()  [unwired: 2 in, 2 out]
            n2614 = property on="Temperature ( Deg C )" class="WFChart (strict)"("XScale.Maximum"=600.0 ("X Scale.Range:Maximum"), "XScale.Minimum"=0.0 ("X Scale.Range:Minimum"), "YScale.Maximum"=100.0 ("Y Scale.Range:Maximum"), "YScale.Minimum"=0.0 ("Y Scale.Range:Minimum")) -> ()  [unwired: 2 in, 2 out]
            n2615 = property on="Humidity ( %RH )" class="WFChart (strict)"("XScale.Maximum"=600.0 ("X Scale.Range:Maximum"), "XScale.Minimum"=0.0 ("X Scale.Range:Minimum"), "YScale.Maximum"=100.0 ("Y Scale.Range:Maximum"), "YScale.Minimum"=0.0 ("Y Scale.Range:Minimum")) -> ()  [unwired: 2 in, 2 out]
            n2616 = property on="Stroke ( mm )" class="WFChart (strict)"("XScale.Maximum"=600.0 ("X Scale.Range:Maximum"), "XScale.Minimum"=0.0 ("X Scale.Range:Minimum"), "YScale.Maximum"=100.0 ("Y Scale.Range:Maximum"), "YScale.Minimum"=0.0 ("Y Scale.Range:Minimum")) -> ()  [unwired: 2 in, 2 out]
            n2617 = property on="Coefficient of Friction" class="WFChart (strict)"("XScale.Maximum"=600.0 ("X Scale.Range:Maximum"), "XScale.Minimum"=0.0 ("X Scale.Range:Minimum"), "YScale.Maximum"=100.0 ("Y Scale.Range:Maximum"), "YScale.Minimum"=0.0 ("Y Scale.Range:Minimum")) -> ()  [unwired: 2 in, 2 out]
            n2618 = property on="Electrical Contact Resistance ( % )" class="WFChart (strict)"("XScale.Minimum"=0.0 ("X Scale.Range:Minimum"), "XScale.Maximum"=600.0 ("X Scale.Range:Maximum"), "YScale.Minimum"=0.0 ("Y Scale.Range:Minimum"), "YScale.Maximum"=100.0 ("Y Scale.Range:Maximum")) -> ()  [unwired: 2 in, 2 out]
            n2619 = property on="Temperature ( Deg C )" class="WFChart (strict)"("XScale.Minimum"=0.0 ("X Scale.Range:Minimum"), "XScale.Maximum"=600.0 ("X Scale.Range:Maximum"), "YScale.Minimum"=0.0 ("Y Scale.Range:Minimum"), "YScale.Maximum"=100.0 ("Y Scale.Range:Maximum")) -> ()  [unwired: 2 in, 2 out]
            n2620 = property on="Coefficient of Friction" class="WFChart (strict)"("XScale.Minimum"=0.0 ("X Scale.Range:Minimum"), "XScale.Maximum"=600.0 ("X Scale.Range:Maximum"), "YScale.Maximum"=1.0 ("X Scale.Range:Minimum"), "YScale.Minimum"=0.0 ("X Scale.Range:Minimum")) -> ()  [unwired: 2 in, 2 out]
            n2621 = property on="Frictional Force ( N )" class="WFChart (strict)"("XScale.Maximum"=600.0 ("X Scale.Range:Maximum"), "XScale.Minimum"=w2700, "YScale.Maximum"=10.0 ("Y Scale.Range:Maximum"), "YScale.Minimum"=w2700) -> ()  [unwired: 2 in, 2 out]
            n2622 = property on="Stroke ( mm )" class="WFChart (strict)"("XScale.Maximum"=600.0 ("X Scale.Range:Maximum"), "XScale.Minimum"=0.0 ("X Scale.Range:Minimum"), "YScale.Maximum"=100.0 ("Y Scale.Range:Maximum"), "YScale.Minimum"=0.0 ("Y Scale.Range:Minimum")) -> ()  [unwired: 2 in, 2 out]
            n2623 = property on="Humidity ( %RH )" class="WFChart (strict)"("XScale.Maximum"=600.0 ("X Scale.Range:Maximum"), "XScale.Minimum"=0.0 ("X Scale.Range:Minimum"), "YScale.Maximum"=100.0 ("Y Scale.Range:Maximum"), "YScale.Minimum"=0.0 ("Y Scale.Range:Minimum")) -> ()  [unwired: 2 in, 2 out]
          }
        }
      }
      frame "Compare Files" {
        # "Elapsed time\ncof\nstroke\nAir temp\nTemp\nHumidity"
        n2624 = case shown="True" "RSTV1 2" {
          frame False {
          }
          frame True {
            n2625 = property on="Humidity ( %RH )" class="XYGraph (strict)"("Y Scale.Display Format:Precision"=u8 0 ("Y Scale.Format & Precision:Precision")) -> ()  [unwired: 2 in, 2 out]
            n2626 = property on="Humidity ( %RH )" class="XYGraph (strict)"("X Scale.Range:Minimum"=0.0, "X Scale.Range:Maximum"=75.0, "Y Scale.Range:Minimum"=48.0, "Y Scale.Range:Maximum"=58.0) -> ()  [unwired: 2 in, 2 out]
          }
        }
        n2627 = case shown="True" "RST CP 2" {
          frame False {
          }
          frame True {
            n2628 = property on="XY Graph 13" class="XYGraph (strict)"("Y Scale.Display Format:Precision"=u8 0 ("Y Scale.Format & Precision:Precision")) -> ()  [unwired: 2 in, 2 out]
            n2629 = property on="XY Graph 13" class="XYGraph (strict)"("X Scale.Range:Minimum"=0.0, "X Scale.Range:Maximum"=75.0, "Y Scale.Range:Minimum"=0.0, "Y Scale.Range:Maximum"=100.0) -> ()  [unwired: 2 in, 2 out]
          }
        }
        n2630 = case shown="True" "RST CP" {
          frame False {
          }
          frame True {
            n2631 = property on="Sample Temperature ( °C )" class="XYGraph (strict)"("Y Scale.Display Format:Precision"=u8 2 ("Y Scale.Format & Precision:Precision")) -> ()  [unwired: 2 in, 2 out]
            n2632 = property on="Sample Temperature ( °C )" class="XYGraph (strict)"("X Scale.Range:Minimum"=0.0, "X Scale.Range:Maximum"=75.0, "Y Scale.Range:Minimum"=58.0, "Y Scale.Range:Maximum"=62.0) -> ()  [unwired: 2 in, 2 out]
          }
        }
        n2633 = case shown="True" "RSTV1 3" {
          frame False {
          }
          frame True {
            n2634 = property on="Air Temperature  ( °C )" class="XYGraph (strict)"("Y Scale.Display Format:Precision"=u8 2 ("Y Scale.Format & Precision:Precision")) -> ()  [unwired: 2 in, 2 out]
            n2635 = property on="Air Temperature  ( °C )" class="XYGraph (strict)"("X Scale.Range:Minimum"=0.0 ("Y Scale.Range:Minimum"), "X Scale.Range:Maximum"=75.0 ("Y Scale.Range:Maximum"), "Y Scale.Range:Minimum"=20.0 ("X Scale.Range:Minimum"), "Y Scale.Range:Maximum"=26.0 ("X Scale.Range:Maximum")) -> ()  [unwired: 2 in, 2 out]
          }
        }
        n2636 = case shown="True" "RSTV1 4" {
          frame False {
          }
          frame True {
            n2637 = property on="Stroke ( mm )" class="XYGraph (strict)"("Y Scale.Display Format:Precision"=u8 2 ("Y Scale.Format & Precision:Precision")) -> ()  [unwired: 2 in, 2 out]
            n2638 = property on="Stroke ( mm )" class="XYGraph (strict)"("X Scale.Range:Minimum"=0.0 ("Y Scale.Range:Maximum"), "X Scale.Range:Maximum"=75.0 ("X Scale.Range:Minimum"), "Y Scale.Range:Minimum"=0.98, "Y Scale.Range:Maximum"=1.02) -> ()  [unwired: 2 in, 2 out]
          }
        }
        n2639 = case shown="True" "rstv2" {
          frame False {
          }
          frame True {
            n2640 = property on="Coefficient Of Friction" class="XYGraph (strict)"("Y Scale.Display Format:Precision"=u8 3 ("Y Scale.Format & Precision:Precision")) -> ()  [unwired: 2 in, 2 out]
            n2641 = property on="Coefficient Of Friction" class="XYGraph (strict)"("X Scale.Range:Minimum"=0.0 ("Y Scale.Range:Maximum"), "X Scale.Range:Maximum"=75.0, "Y Scale.Range:Minimum"=0.0, "Y Scale.Range:Maximum"=1.0 ("X Scale.Range:Minimum")) -> ()  [unwired: 2 in, 2 out]
          }
        }
        n2642 = case shown="True" "RST CP 3" {
          frame False {
          }
          frame True {
            n2643 = property on="Air Temp ( °C ) vs Humidity ( % RH )" class="XYGraph (strict)"("X Scale.Range:Minimum"=18.0, "X Scale.Range:Maximum"=28.0 ("X Scale.Range:Minimum"), "Y Scale.Range:Minimum"=30.0 ("X Scale.Range:Minimum"), "Y Scale.Range:Maximum"=70.0 ("X Scale.Range:Minimum")) -> ()  [unwired: 2 in, 2 out]
          }
        }
        n2644 = case shown="True" "OPEN 1" {
          frame False {
          }
          frame True {
            (unwired) 0  # existing file
            w3419 = "Choose a datalog file to open"  # prompt
            n2645 = local write "OPEN 1"(FALSE ("OPEN 1")) -> ()
            n2646 = String To Path(string="C:\\LAB-IQ\\Data\\") -> (path=w3404:path)
            n2647 = File Dialog(6:"*.dgf" ("pattern"), 7:w3419, 11:w3404) -> (0:w3402:errorcluster, 3:w3410:path)  [unwired: 4 in, 2 out]
            n2648 = Unbundle(w3402) -> ()  [unwired: 3 out]
            n2649 = Strip Path(path=w3410) -> (name=w3409:string)  [unwired: 1 out]
            n2650 = Path To String(path=w3410) -> (string=w3405:string)
            "string1" <- w3405
            n2651 = Match Pattern(string=w3409, regular expression=".dgf") -> (before substring=→"String Control":string)  [unwired: 1 in, 3 out]
            n2652 = Match Pattern(string=w3405, regular expression=".dgf" ("substring (\"\")")) -> (before substring=w3415:string)  [unwired: 1 in, 3 out]
            n2653 = Concatenate Strings(w3415, ".duf" ("Substring")) -> (w3411:string)
            n2654 = String To Path(string=w3411) -> (path=w3416:path)
            n2655 = call <vilib>:"Read Characters From File.vi"("file path (dialog if empty)"=w3416, "start of read offset (chars.:0)"=60 ("start of read offset (chars.: 0)")) -> ("character string"=→"String Control 2":string)  [unwired: 4 in, 3 out]
          }
        }
        n2656 = case shown="True" "OPEN 2" {
          frame False {
          }
          frame True {
            (unwired) 0  # existing file
            w3437 = "Choose a datalog file to open"  # prompt
            n2657 = local write "OPEN 2"(FALSE ("OPEN 1")) -> ()
            n2658 = String To Path(string="C:\\LAB-IQ\\Data\\") -> (path=w3422:path)
            n2659 = File Dialog(6:"*.dgf" ("pattern"), 7:w3437, 11:w3422) -> (0:w3420:errorcluster, 3:w3428:path)  [unwired: 4 in, 2 out]
            n2660 = Unbundle(w3420) -> ()  [unwired: 3 out]
            n2661 = Strip Path(path=w3428) -> (name=w3426:string)  [unwired: 1 out]
            n2662 = Path To String(path=w3428) -> (string=w3423:string)
            "string1 2" <- w3423
            n2663 = Match Pattern(string=w3426, regular expression=".dgf") -> (before substring=→"String Control 3":string)  [unwired: 1 in, 3 out]
            n2664 = Match Pattern(string=w3423, regular expression=".dgf" ("substring (\"\")")) -> (before substring=w3434:string)  [unwired: 1 in, 3 out]
            n2665 = Concatenate Strings(w3434, ".duf" ("Substring")) -> (w3431:string)
            n2666 = String To Path(string=w3431) -> (path=w3429:path)
            n2667 = call <vilib>:"Read Characters From File.vi"("file path (dialog if empty)"=w3429, "start of read offset (chars.:0)"=60 ("start of read offset (chars.: 0)")) -> ("character string"=→"String Control 4":string)  [unwired: 4 in, 3 out]
          }
        }
        n2668 = case shown="True" "OPEN 3" {
          frame False {
          }
          frame True {
            (unwired) 0  # existing file
            w3455 = "Choose a datalog file to open"  # prompt
            n2669 = local write "OPEN 3"(FALSE ("OPEN 1")) -> ()
            n2670 = String To Path(string="C:\\LAB-IQ\\Data\\") -> (path=w3440:path)
            n2671 = File Dialog(6:"*.dgf" ("pattern"), 7:w3455, 11:w3440) -> (0:w3438:errorcluster, 3:w3446:path)  [unwired: 4 in, 2 out]
            n2672 = Unbundle(w3438) -> ()  [unwired: 3 out]
            n2673 = Strip Path(path=w3446) -> (name=w3444:string)  [unwired: 1 out]
            n2674 = Path To String(path=w3446) -> (string=w3441:string)
            "string1 3" <- w3441
            n2675 = Match Pattern(string=w3444, regular expression=".dgf") -> (before substring=→"String Control 5":string)  [unwired: 1 in, 3 out]
            n2676 = Match Pattern(string=w3441, regular expression=".dgf" ("substring (\"\")")) -> (before substring=w3451:string)  [unwired: 1 in, 3 out]
            n2677 = Concatenate Strings(w3451, ".duf" ("Substring")) -> (w3448:string)
            n2678 = String To Path(string=w3448) -> (path=w3452:path)
            n2679 = call <vilib>:"Read Characters From File.vi"("file path (dialog if empty)"=w3452, "start of read offset (chars.:0)"=60 ("start of read offset (chars.: 0)")) -> ("character string"=→"String Control 6":string)  [unwired: 4 in, 3 out]
          }
        }
        n2680 = case shown="True" "OPEN 4" {
          frame False {
          }
          frame True {
            (unwired) 0  # existing file
            w3473 = "Choose a datalog file to open"  # prompt
            n2681 = local write "OPEN 4"(FALSE ("OPEN 1")) -> ()
            n2682 = String To Path(string="C:\\LAB-IQ\\Data\\") -> (path=w3458:path)
            n2683 = File Dialog(6:"*.dgf" ("pattern"), 7:w3473, 11:w3458) -> (0:w3456:errorcluster, 3:w3464:path)  [unwired: 4 in, 2 out]
            n2684 = Unbundle(w3456) -> ()  [unwired: 3 out]
            n2685 = Strip Path(path=w3464) -> (name=w3462:string)  [unwired: 1 out]
            n2686 = Path To String(path=w3464) -> (string=w3459:string)
            "string1 4" <- w3459
            n2687 = Match Pattern(string=w3462, regular expression=".dgf") -> (before substring=→"String Control 7":string)  [unwired: 1 in, 3 out]
            n2688 = Match Pattern(string=w3459, regular expression=".dgf" ("substring (\"\")")) -> (before substring=w3469:string)  [unwired: 1 in, 3 out]
            n2689 = Concatenate Strings(w3469, ".duf" ("Substring")) -> (w3466:string)
            n2690 = String To Path(string=w3466) -> (path=w3470:path)
            n2691 = call <vilib>:"Read Characters From File.vi"("file path (dialog if empty)"=w3470, "start of read offset (chars.:0)"=60 ("start of read offset (chars.: 0)")) -> ("character string"=→"String Control 8":string)  [unwired: 4 in, 3 out]
          }
        }
      }
      frame "About" {
        # "Elapsed time\ncof\nstroke\nmean pos\nTemp\nHumidity"
        n2692 = disable-structure shown="Disabled" {
          frame Disabled {
            n2693 = case shown="True" "Export" {
              frame False {
              }
              frame True {
                w3495 = "                                      " ("string")
                w3497 = "\r"
                (unwired) i16 6 ("width (-)")
                w3574 = "\r"
                w3506 = "\r"
                n2694 = local write "Export"(FALSE ("Export")) -> ()
                n2695 = local read "String 29"() -> (w3543:string)
                n2696 = local read "String 34"() -> (w3531:string)
                n2697 = local read "String 35"() -> (w3526:string)
                n2698 = local read "String 37"() -> (w3522:string)
                n2699 = local read "String 36"() -> (w3519:string)
                n2700 = local read "String 38"() -> (w3516:string)
                n2701 = local read "String 39"() -> (w3513:string)
                n2702 = Match Pattern(string=w3543, regular expression=".dwm") -> (before substring=w3539:string)  [unwired: 1 in, 3 out]
                "before substring" <- w3539
                n2703 = local read "S 38"() -> (w3534:string)
                n2704 = local read "S 39"() -> (w3527:string)
                n2705 = local read "Temperature before test 2"() -> (w3563:dbl)
                n2706 = local read "Temperature after test 2"() -> (w3568:dbl)
                n2707 = local read "Humidity before test 2"() -> (w3549:dbl)
                n2708 = local read "Humidity after test 2"() -> (w3564:dbl)
                n2709 = local read "MWSD 2"() -> (w3560:dbl)
                n2710 = local read "WS1.4 2"() -> (w3576:dbl)
                n2711 = local read "HCF 2"() -> (w3572:dbl)
                n2712 = local read "AVP 2"() -> (w3561:dbl)
                n2713 = Concatenate Strings("1," ("string"), w3534) -> (w3533:string)
                n2714 = Concatenate Strings("2," ("string"), w3531) -> (w3530:string)
                n2715 = Concatenate Strings("3," ("string"), w3527) -> (w3529:string)
                n2716 = Concatenate Strings("4," ("string"), w3526) -> (w3525:string)
                n2717 = Concatenate Strings("5," ("string"), w3522) -> (w3523:string)
                n2718 = Concatenate Strings("6," ("string"), w3519) -> (w3520:string)
                n2719 = Concatenate Strings("7," ("string"), w3516) -> (w3517:string)
                n2720 = Concatenate Strings("8," ("string"), w3513) -> (w3514:string)
                n2721 = local read "Sample ID"() -> (w3581:string)
                n2722 = case shown="\"xlx\"" "Select File Type" {
                  tunnel: w3539 -> [w3584 w3586 w3588]
                  tunnel: [w3582 w3587 w3589] -> w3538
                  frame "xlx" {
                    n2723 = Concatenate Strings(w3584, ".xls" ("string")) -> (w3582:string)
                  }
                  frame "csv" {
                    n2724 = Concatenate Strings(w3586, ".csv" ("string")) -> (w3587:string)
                  }
                  frame "txt" {
